vi "report_REsult_to_string.vi"(8 "error in (no error)":errorcluster, 11 "Array in":string[][](array[string])) -> (0 "error out":errorcluster, 3 "Array out":string[][](array[string]))   [LabVIEW 2017]
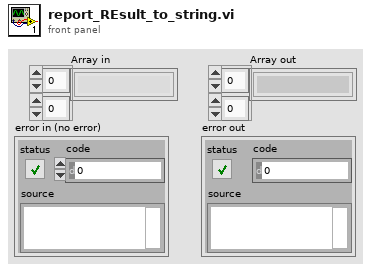
[diagram p1: front panel]
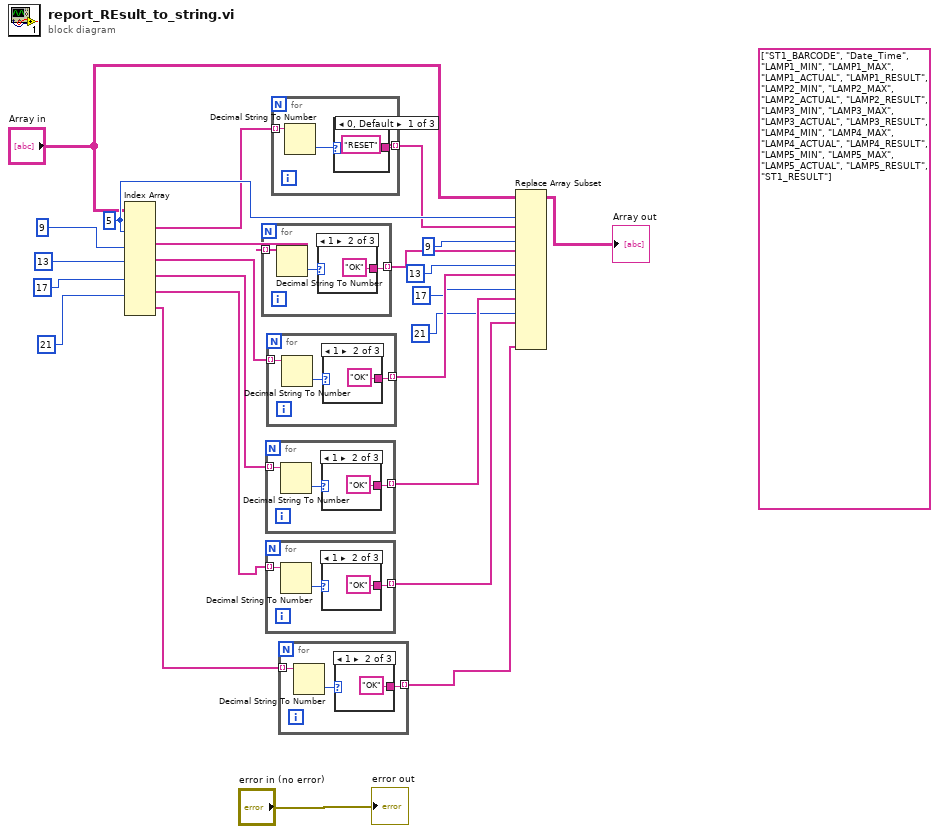
[diagram p0: block diagram]
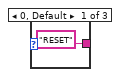
[diagram p2: hidden frame]
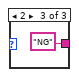
[diagram p3: hidden frame]
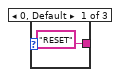
[diagram p4: hidden frame]
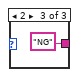
[diagram p5: hidden frame]
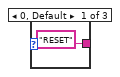
[diagram p6: hidden frame]
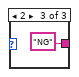
[diagram p7: hidden frame]
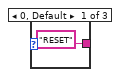
[diagram p8: hidden frame]
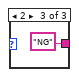
[diagram p9: hidden frame]
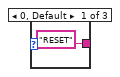
[diagram p10: hidden frame]
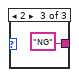
[diagram p11: hidden frame]
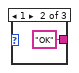
[diagram p12: hidden frame]
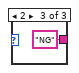
[diagram p13: hidden frame]
diagram:
  (unwired) string[] ["ST1_BARCODE", "Date_Time", "LAMP1_MIN", "LAMP1_MAX", "LAMP1_ACTUAL", "LAMP1_RESULT", "LAMP2_MIN", "LAMP2_MAX", "LAMP2_ACTUAL", "LAMP2_RESULT", "LAMP3_MIN", "LAMP3_MAX", "LAMP3_ACTUAL", "LAMP3_RESULT", "LAMP4_MIN", "LAMP4_MAX", "LAMP4_ACTUAL", "LAMP4_RESULT", "LAMP5_MIN", "LAMP5_MAX", "LAMP5_ACTUAL", "LAMP5_RESULT", "ST1_RESULT"]
  w19 = 5 ("index (row)")
  n1 = Index Array(array="Array in", index (col) #1=w19, index (col) #2=9 ("index (row)"), index (col) #3=13 ("index (row)"), index (col) #4=17 ("index (row)"), index (col) #5=21 ("index (row)")) -> (element #1=w16:string[], element #2=w22:string[], element #3=w13:string[], element #4=w9:string[], element #5=w4:string[], element #6=w1:string[])  [unwired: 7 in]
  n2 = for {
    tunnel: [w26] -> w24 mode=indexing
    tunnel: w22 -> [w25] mode=indexing
    n3 = Decimal String To Number(string=w25) -> (number=w27:i32)  [unwired: 2 in, 1 out]
    n4 = case shown="1" w27 {
      tunnel: ["RESET" "OK" "NG"] -> w26
      frame 0, Default {
      }
      frame 1 {
      }
      frame 2 {
      }
    }
  }
  n5 = for {
    tunnel: [w32] -> w8 mode=indexing
    tunnel: w9 -> [w31] mode=indexing
    n6 = Decimal String To Number(string=w31) -> (number=w33:i32)  [unwired: 2 in, 1 out]
    n7 = case shown="1" w33 {
      tunnel: ["RESET" "OK" "NG"] -> w32
      frame 0, Default {
      }
      frame 1 {
      }
      frame 2 {
      }
    }
  }
  n8 = for {
    tunnel: [w38] -> w6 mode=indexing
    tunnel: w4 -> [w37] mode=indexing
    n9 = Decimal String To Number(string=w37) -> (number=w39:i32)  [unwired: 2 in, 1 out]
    n10 = case shown="1" w39 {
      tunnel: ["RESET" "OK" "NG"] -> w38
      frame 0, Default {
      }
      frame 1 {
      }
      frame 2 {
      }
    }
  }
  n11 = for {
    tunnel: [w44] -> w11 mode=indexing
    tunnel: w13 -> [w43] mode=indexing
    n12 = Decimal String To Number(string=w43) -> (number=w45:i32)  [unwired: 2 in, 1 out]
    n13 = case shown="1" w45 {
      tunnel: ["RESET" "OK" "NG"] -> w44
      frame 0, Default {
      }
      frame 1 {
      }
      frame 2 {
      }
    }
  }
  n14 = for {
    tunnel: [w50] -> w18 mode=indexing
    tunnel: w16 -> [w49] mode=indexing
    n15 = Decimal String To Number(string=w49) -> (number=w51:i32)  [unwired: 2 in, 1 out]
    n16 = case shown="0, Default" w51 {
      tunnel: ["RESET" "OK" "NG"] -> w50
      frame 0, Default {
      }
      frame 1 {
      }
      frame 2 {
      }
    }
  }
  n17 = for {
    tunnel: [w56] -> w2 mode=indexing
    tunnel: w1 -> [w55] mode=indexing
    n18 = Decimal String To Number(string=w55) -> (number=w57:i32)  [unwired: 2 in, 1 out]
    n19 = case shown="1" w57 {
      tunnel: ["RESET" "OK" "NG"] -> w56
      frame 0, Default {
      }
      frame 1 {
      }
      frame 2 {
      }
    }
  }
  n20 = Replace Array Subset(array="Array in", new element #1=w18, index (col) #1=w19, new element #2=w24, index (col) #2=9 ("index (row)"), new element #3=w11, index (col) #3=13 ("index (row)"), new element #4=w8, index (col) #4=17 ("index (row)"), new element #5=w6, index (col) #5=21 ("index (row)"), new element #6=w2) -> (→"Array out":string[][])  [unwired: 7 in]
  "error out" <- "error in (no error)"
